vi "Autonomous Independent.vi"   [LabVIEW 2011]
doc: "This VI is called when autonomous begins, and will automatically be terminated when autonomous ends. You can carry out timed or sensor driven robot movement independently without needing to return to the caller."
uses:
  <vilib>/Rock Robotics/WPI/Solenoid/WPI_SolenoidValue.ctl
  Robot Global Data.vi
  <vilib>/Rock Robotics/WPI/Solenoid/WPI_SolenoidSetEnum.vi
types:
  T1 = typedef "WPI_RobotDriveDevRef.ctl" = cluster{"DevStatus":errorcluster, "Motors[]":T2[], "Square Inputs":bool, "Max Output":dbl, "Isochronous":bool}
  T2 = typedef "WPI_MotorControlDeviceRef.ctl" = cluster{"DeviceStatus":errorcluster, "Type":enum16{"PWM", "CAN"}, "PWM":cluster{"Digital Module":T3, "PWM Channel":T4, "DeadBand":T5}, "CAN":cluster{"Device Number":u8, "Control Mode":T6, "Semaphore":T7, "Max Vout":dbl}, "Invert":bool, "TransformRef":T8, "InvTransformRef":T8}
  T3 = typedef "FPGA_TypedefDigitalModule.ctl" = enum16{"Digital Module 1", "Digital Module 2"}
  T4 = typedef "FPGA_DIOPWMChannel.ctl" = enum8{"PWM 1", "PWM 2", "PWM 3", "PWM 4", "PWM 5", "PWM 6", "PWM 7", "PWM 8", "PWM 9", "PWM 10", "Invalid"}
  T5 = typedef "WPI_PWMDeadband.ctl" = cluster{"Name":string, "maxPositivePwm":i32, "minPositivePwm":i32, "centerPwm":i32, "maxNegativePwm":i32, "minNegativePwm":i32, "angularRange":u16}
  T6 = typedef "WPI_CANJaguar_ControlMode.ctl" = enum8{"Percent VBus", "Current", "Speed", "Position", "Voltage"}
  T7 = typedef "Semaphore RefNum" = refnum<k1>
  T8 = typedef "WPI_PWMTransform_ConPane.ctl" = refnum<vi>
  T9 = typedef "Autonomous Data.ctl" = cluster{"Auto Mode":enum16{"Do Nothing", "Shoot From Key", "Shoot From Key Center, Bridge", "Shoot From Key, Feed", "Shoot From Key, Drive Forward", "Fender From Center", "Fender From Right", "Fender From Left"}, "Delay (s)":dbl}
  T10 = typedef "WPI_GyroDevRef.ctl" = cluster{"DevStatus":errorcluster, "Analog Module":T11, "Analog Channel":T12, "Offset":dbl, "Gain (VoltsPerDegree/Second)":dbl}
  T11 = typedef "FPGA_TypedefAnalogModule.ctl" = enum16{"Analog Module 1", "Analog Module 2"}
  T12 = typedef "FPGA_AIChannel.ctl" = enum8{"AI 1", "AI 2", "AI 3", "AI 4", "AI 5", "AI 6", "AI 7", "AI 8", "Invalid"}
  T13 = enum16{"Do Nothing", "Shoot From Key", "Shoot From Key Center, Bridge", "Shoot From Key, Feed", "Shoot From Key, Drive Forward", "Fender From Center", "Fender From Right", "Fender From Left"}
  T14 = typedef "WPI_SolenoidValue.ctl" = enum16{"Off", "On", "Forward", "Reverse"}
  T15 = typedef "Position Typedef.ctl" = cluster{"X":dbl, "Y":dbl, "Heading":dbl}
  T16 = typedef "WPI_SolenoidDevRef.ctl" = cluster{"DevStatus":errorcluster, "Solenoid Module":T17, "Forward Solenoid Channel":T18, "Reverse Solenoid Channel":T18}
  T17 = typedef "FPGA_TypedefSolenoidModule.ctl" = enum16{"Solenoid Module 1", "Solenoid Module 2"}
  T18 = typedef "WPI_SolenoidChannel.ctl" = enum8{"Solenoid 1", "Solenoid 2", "Solenoid 3", "Solenoid 4", "Solenoid 5", "Solenoid 6", "Solenoid 7", "Solenoid 8", "Invalid"}
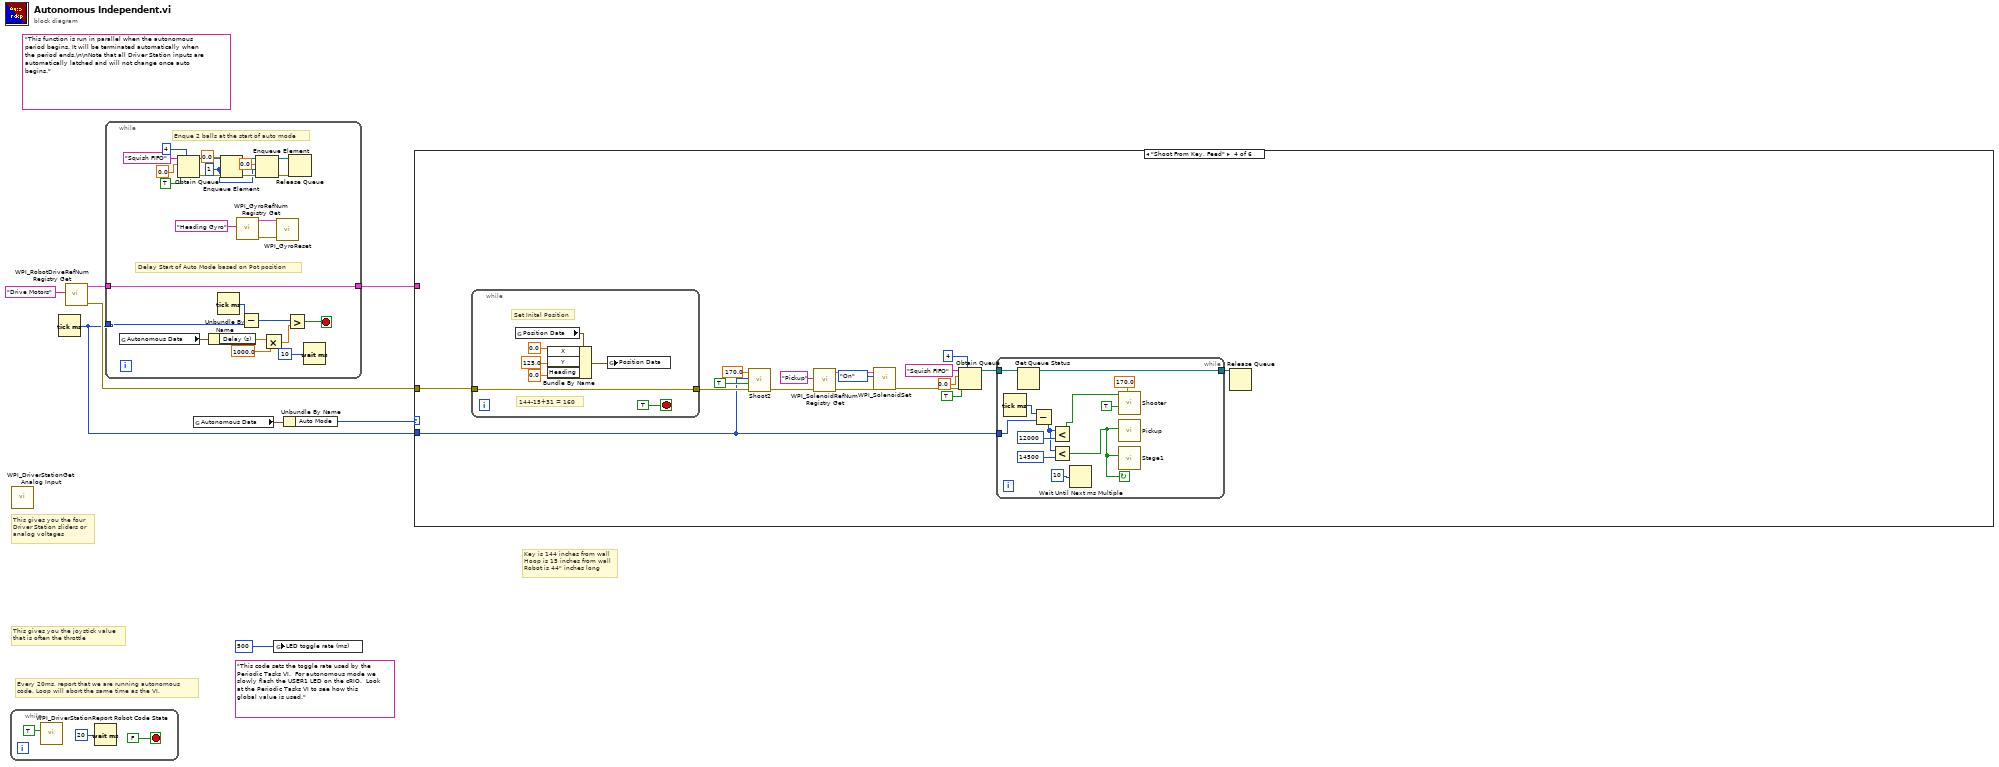
[diagram p0: block diagram]
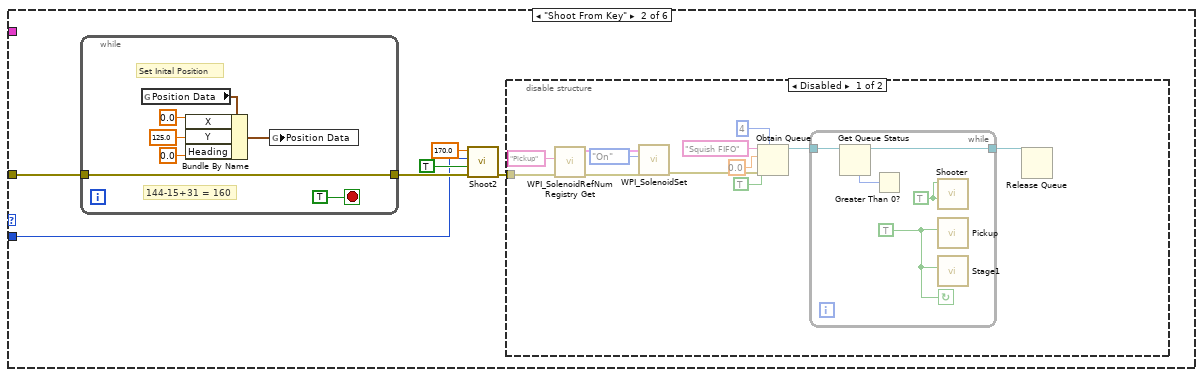
[diagram p3: hidden frame]
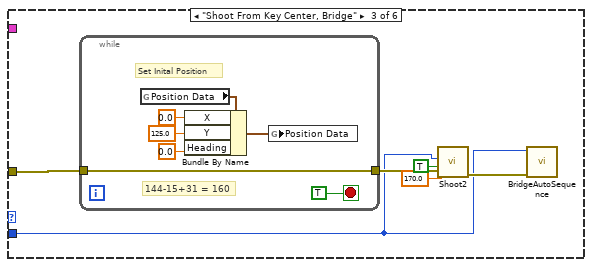
[diagram p5: hidden frame]
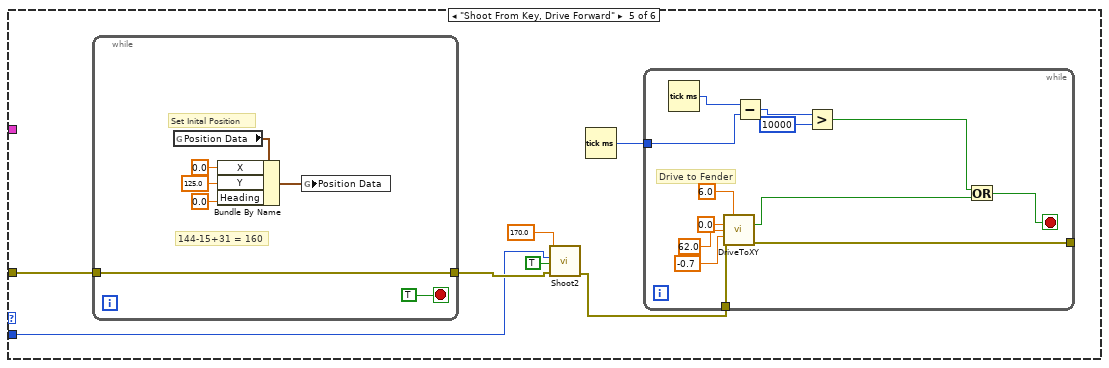
[diagram p6: hidden frame]
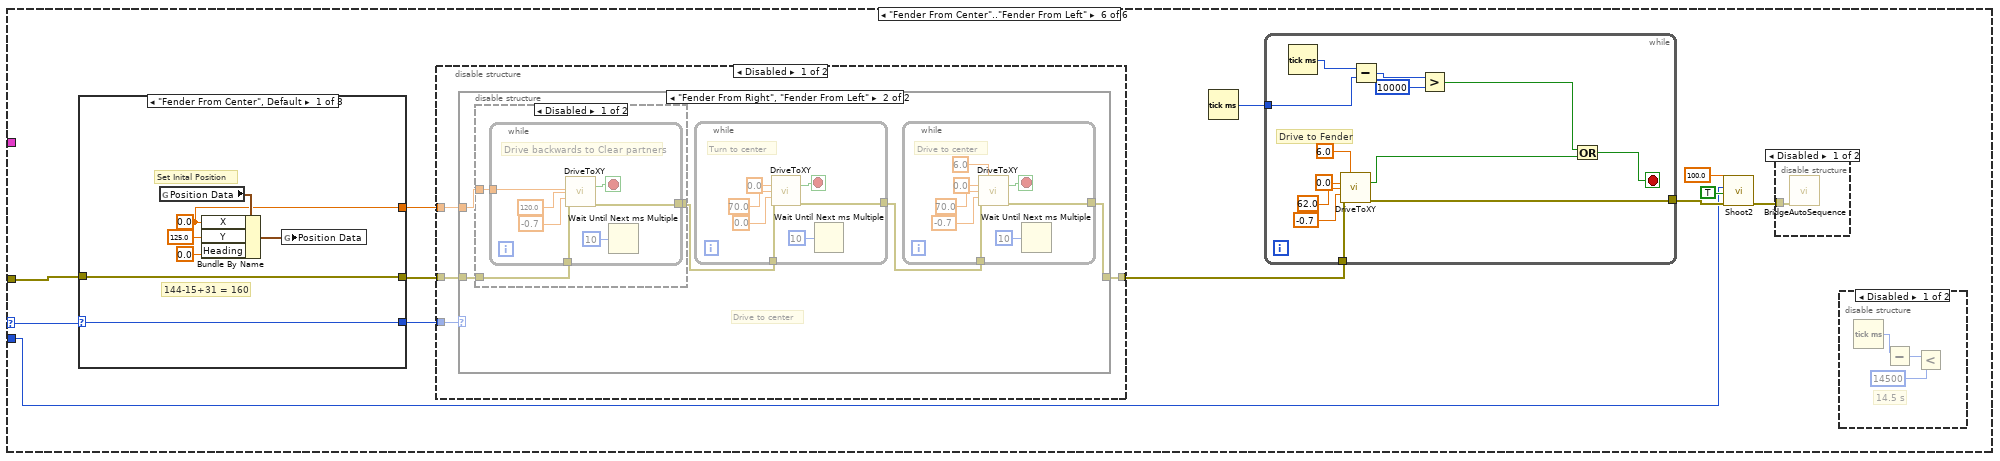
[diagram p7: hidden frame]
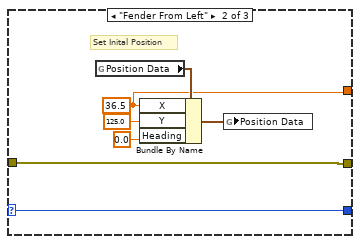
[diagram p13: hidden frame]
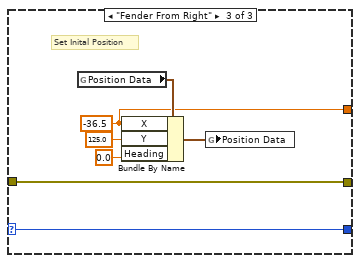
[diagram p14: hidden frame]
diagram:
  (unwired) "This code sets the toggle rate used by the Periodic Tasks VI.  For autonomous mode we slowly flash the USER1 LED on the cRIO.  Look at the Periodic Tasks VI to see how this global value is used."
  (unwired) "This function is run in parallel when the autonomous period begins. It will be terminated automatically when the period ends.\n\nNote that all Driver Station inputs are automatically latched and will not change once auto begins."
  # "Key is 144 inches from wall\nHoop is 15 inches from wall\nRobot is 44\" inches long"
  # "Every 20ms, report that we are running autonomous\ncode. Loop will abort the same time as the VI."
  # "This gives you the joystick value\nthat is often the throttle"
  # "This gives you the four\nDriver Station sliders or\nanalog voltages"
  n1 = while {
    stop <- FALSE stop-if-true
    n2 = call <vilib>:"WPI_DriverStationReport Robot Code State.vi"("Autonomous"=TRUE) -> ()  [unwired: 10 in, 1 out]
    n3 = Wait (ms)(milliseconds to wait=u32 20) -> ()  [unwired: 1 out]
  }
  n4 = call <vilib>:"WPI_DriverStationGet Analog Input.vi"() -> ()  [unwired: 12 out]
  n5 = Tick Count (ms)() -> (millisecond timer value=w1:u32)
  n6 = call <vilib>:"WPI_RobotDriveRefNum Registry Get.vi"("refnum name"="Drive Motors") -> ("error out"=w2:errorcluster, "RobotDriveDevRef"=w6:T1)  [unwired: 1 in, 8 out]
  n7 = while {
    tunnel: w1 -> [w36]
    tunnel: w6 -> [w33]
    tunnel: [w33] -> w3
    stop <- w35 stop-if-true
    w14 = 1 ("timeout in ms (-1)")
    # "Enque 2 balls at the start of auto mode"
    # "Delay Start of Auto Mode based on Pot position"
    n8 = global read "Robot Global Data.vi" "Autonomous Data"() -> (w31:T9)
    n9 = Obtain Queue(max queue size (-1, unlimited)=4, name (unnamed)="Squish FIFO", element data type=sgl 0.0 ("Voltage"), create if not found? (T)=TRUE) -> (queue out=w21:refnum<queue>, error out=w22:errorcluster)  [unwired: 1 in, 1 out]
    n10 = Unbundle By Name(w31) -> ("Delay (s)"=w29:dbl)
    n11 = Tick Count (ms)() -> (millisecond timer value=w32:u32)
    n12 = Enqueue Element(queue=w21, element=sgl 0.0, timeout in ms (-1)=w14, error in (no error)=w22) -> (queue out=w17:refnum<queue>, error out=w16:errorcluster)  [unwired: 1 out]
    n13 = call <vilib>:"WPI_GyroRefNum Registry Get.vi"("refnum name"="Heading Gyro") -> ("error out"=w26:errorcluster, "GyroDevRef"=w25:T10)  [unwired: 1 in, 8 out]
    n14 = Subtract(x=w32, y=w36) -> (x-y=w37:u32)
    n15 = Enqueue Element(queue=w17, element=sgl 0.0, timeout in ms (-1)=w14, error in (no error)=w16) -> (queue out=w12:refnum<queue>, error out=w13:errorcluster)  [unwired: 1 out]
    n16 = Multiply(x=w29, y=1000.0) -> (x*y=w30:dbl)
    n17 = call <vilib>:"WPI_GyroReset.vi"("error in (no error)"=w26, "GyroDevRef"=w25) -> ()  [unwired: 8 in, 2 out]
    n18 = Greater?(x=w37, y=w30) -> (0:w35:bool)
    n19 = Release Queue(queue=w12, error in (no error)=w13) -> ()  [unwired: 1 in, 3 out]
    n20 = Wait (ms)(milliseconds to wait=u32 10) -> ()  [unwired: 1 out]
  }
  n21 = global read "Robot Global Data.vi" "Autonomous Data"() -> (w5:T9)
  n22 = global write "Robot Global Data.vi" "LED toggle rate (ms)"(u32 500 ("LED ms toggle rate")) -> ()
  n23 = Unbundle By Name(w5) -> ("Auto Mode"=w4:T13)
  n24 = case shown="\"Shoot From Key, Feed\"" w4 {
    selector: w4 -> [_ _ _ _ _ w155]
    tunnel: w3 -> [_ _ _ _ _ _]
    tunnel: w2 -> [_ w43 w73 w94 w121 w154]
    tunnel: w1 -> [_ w39 w69 w81 w117 w145]
    frame "Do Nothing", Default {
    }
    frame "Shoot From Key" {
      n25 = while {
        tunnel: w43 -> [w64]
        tunnel: [w64] -> w42
        stop <- TRUE stop-if-true
        # "144-15+31 = 160"
        # "Set Inital Position"
        n26 = global read "Robot Global Data.vi" "Position Data"() -> (w67:T15)
        n27 = Bundle By Name(cluster=w67, "X"=0.0, "Y"=125.0, "Heading"=0.0) -> (w66:T15)
        n28 = global write "Robot Global Data.vi" "Position Data"(w66) -> ()
      }
      n29 = call "Shoot2.vi"("error in (no error)"=w42, "Use Camera"=TRUE, "Auto Start"=w39, "Distance"=170.0) -> ("error out"=w41:errorcluster)  [unwired: 7 in]
      n30 = disable-structure shown="Disabled" {
        disable-tunnel: w41 -> [w47 _]
        frame Disabled {
          n31 = call <vilib>:"WPI_SolenoidRefNum Registry Get.vi"("error in (no error)"=w47, "refnum name"="Pickup") -> ("error out"=w51:errorcluster, "SolenoidDevRef"=w49:T16)  [unwired: 8 in]
          n32 = call-poly <vilib>:"WPI_SolenoidSet.vi"("error in (no error)"=w51, "Value"=WPI_SolenoidValue."On", "SolenoidDevRef"=w49) -> ("error out"=w46:errorcluster)  [unwired: 7 in, 1 out]
          n33 = Obtain Queue(max queue size (-1, unlimited)=4, name (unnamed)="Squish FIFO", element data type=sgl 0.0 ("Voltage"), create if not found? (T)=TRUE, error in (no error)=w46) -> (queue out=w52:refnum<queue>)  [unwired: 2 out]
          n34 = while {
            tunnel: w52 -> [w58]
            tunnel: [w57] -> w45
            stop <- w60 continue-if-true
            w56 = TRUE ("Use Camera")
            w60 = TRUE ("Fire")
            n35 = Get Queue Status(queue=w58) -> (queue out=w57:refnum<queue>, # elements in queue=w59:i32)  [unwired: 2 in, 6 out]
            n36 = Greater Than 0?(x=w59) -> ()  [unwired: 1 out]
            n37 = call "Shooter.vi"("Use Camera"=w56, "Fire"=w56) -> ()  [unwired: 8 in, 2 out]
            n38 = call "Pickup.vi"("On?"=w60) -> ()  [unwired: 11 in]
            n39 = call "Stage1.vi"("On?"=w60) -> ()  [unwired: 11 in]
          }
          n40 = Release Queue(queue=w45) -> ()  [unwired: 2 in, 3 out]
        }
        frame Enabled {
        }
      }
    }
    frame "Shoot From Key Center, Bridge" {
      n41 = while {
        tunnel: w73 -> [w77]
        tunnel: [w77] -> w72
        stop <- TRUE stop-if-true
        # "144-15+31 = 160"
        # "Set Inital Position"
        n42 = global read "Robot Global Data.vi" "Position Data"() -> (w80:T15)
        n43 = Bundle By Name(cluster=w80, "X"=0.0, "Y"=125.0, "Heading"=0.0) -> (w79:T15)
        n44 = global write "Robot Global Data.vi" "Position Data"(w79) -> ()
      }
      n45 = call "Shoot2.vi"("error in (no error)"=w72, "Use Camera"=TRUE, "Auto Start"=w69, "Distance"=170.0) -> ("error out"=w71:errorcluster)  [unwired: 7 in]
      n46 = call "BridgeAutoSequence.vi"("error in (no error)"=w71, "Auto Start"=w69) -> ()  [unwired: 10 in]
    }
    frame "Shoot From Key, Feed" {
      n47 = while {
        tunnel: w94 -> [w113]
        tunnel: [w113] -> w97
        stop <- TRUE stop-if-true
        # "144-15+31 = 160"
        # "Set Inital Position"
        n48 = global read "Robot Global Data.vi" "Position Data"() -> (w116:T15)
        n49 = Bundle By Name(cluster=w116, "X"=0.0, "Y"=125.0, "Heading"=0.0) -> (w115:T15)
        n50 = global write "Robot Global Data.vi" "Position Data"(w115) -> ()
      }
      n51 = call "Shoot2.vi"("error in (no error)"=w97, "Use Camera"=TRUE, "Auto Start"=w81, "Distance"=170.0) -> ("error out"=w82:errorcluster)  [unwired: 7 in]
      n52 = call <vilib>:"WPI_SolenoidRefNum Registry Get.vi"("error in (no error)"=w82, "refnum name"="Pickup") -> ("error out"=w89:errorcluster, "SolenoidDevRef"=w87:T16)  [unwired: 8 in]
      n53 = call-poly <vilib>:"WPI_SolenoidSet.vi"("error in (no error)"=w89, "Value"=WPI_SolenoidValue."On", "SolenoidDevRef"=w87) -> ("error out"=w85:errorcluster)  [unwired: 7 in, 1 out]
      n54 = Obtain Queue(max queue size (-1, unlimited)=4, name (unnamed)="Squish FIFO", element data type=sgl 0.0 ("Voltage"), create if not found? (T)=TRUE, error in (no error)=w85) -> (queue out=w90:refnum<queue>)  [unwired: 2 out]
      n55 = while {
        tunnel: w90 -> [w109]
        tunnel: [w108] -> w84
        tunnel: w81 -> [w103]
        stop <- w98 continue-if-true
        n56 = Tick Count (ms)() -> (millisecond timer value=w104:u32)
        n57 = Get Queue Status(queue=w109) -> (queue out=w108:refnum<queue>)  [unwired: 2 in, 7 out]
        n58 = Subtract(x=w104, y=w103) -> (x-y=w100:u32)
        n59 = Less?(x=w100, y=u32 12000) -> (x < y?=w101:bool)
        n60 = Less?(x=w100, y=u32 14500) -> (x < y?=w98:bool)
        n61 = Wait Until Next ms Multiple(millisecond multiple=u32 10) -> ()  [unwired: 1 out]
        n62 = call "Shooter.vi"("Distance"=170.0, "Use Camera"=TRUE, "Fire"=w101) -> ()  [unwired: 7 in, 2 out]
        n63 = call "Pickup.vi"("On?"=w98) -> ()  [unwired: 11 in]
        n64 = call "Stage1.vi"("On?"=w98) -> ()  [unwired: 11 in]
      }
      n65 = Release Queue(queue=w84) -> ()  [unwired: 2 in, 3 out]
    }
    frame "Shoot From Key, Drive Forward" {
      n66 = while {
        tunnel: w121 -> [w124]
        tunnel: [w124] -> w119
        stop <- TRUE stop-if-true
        # "144-15+31 = 160"
        # "Set Inital Position"
        n67 = global read "Robot Global Data.vi" "Position Data"() -> (w129:T15)
        n68 = Bundle By Name(cluster=w129, "X"=0.0, "Y"=125.0, "Heading"=0.0) -> (w128:T15)
        n69 = global write "Robot Global Data.vi" "Position Data"(w128) -> ()
      }
      n70 = call "Shoot2.vi"("error in (no error)"=w119, "Use Camera"=TRUE, "Auto Start"=w117, "Distance"=170.0) -> ("error out"=w118:errorcluster)  [unwired: 7 in]
      n71 = Tick Count (ms)() -> (millisecond timer value=w122:u32)
      n72 = while {
        tunnel: [w141] -> _
        tunnel: w118 -> [w140]
        tunnel: w122 -> [w137]
        stop <- w132 stop-if-true
        # "Drive to Fender"
        n73 = Tick Count (ms)() -> (millisecond timer value=w138:u32)
        n74 = call "DriveToXY.vi"("Drive Margin"=6.0, "X Target"=0.0, "Y Target"=62.0, "Speed"=-0.7, "error in"=w140) -> ("At Target"=w134:bool, "error out"=w141:errorcluster)  [unwired: 8 in, 1 out]
        n75 = Subtract(x=w138, y=w137) -> (x-y=w136:u32)
        n76 = Greater?(x=w136, y=u32 10000) -> (0:w133:bool)
        n77 = Or(x=w133, y=w134) -> (x .or. y?=w132:bool)
      }
    }
    frame "Fender From Center".."Fender From Left" {
      n78 = case shown="\"Fender From Center\", Default" w155 {
        selector: w155 -> [w208 w215 w223]
        tunnel: w154 -> [w210 w217 w224]
        tunnel: [w210 w217 w224] -> w153
        tunnel: [w209 w216 w222] -> w152
        tunnel: [w208 w215 w223] -> w150
        frame "Fender From Center", Default {
          w209 = 0.0 ("X")
          # "144-15+31 = 160"
          # "Set Inital Position"
          n79 = global read "Robot Global Data.vi" "Position Data"() -> (w214:T15)
          n80 = Bundle By Name(cluster=w214, "X"=w209, "Y"=125.0, "Heading"=0.0) -> (w213:T15)
          n81 = global write "Robot Global Data.vi" "Position Data"(w213) -> ()
        }
        frame "Fender From Left" {
          w216 = 36.5 ("X")
          # "Set Inital Position"
          n82 = global read "Robot Global Data.vi" "Position Data"() -> (w221:T15)
          n83 = Bundle By Name(cluster=w221, "X"=w216, "Y"=125.0, "Heading"=0.0) -> (w220:T15)
          n84 = global write "Robot Global Data.vi" "Position Data"(w220) -> ()
        }
        frame "Fender From Right" {
          w222 = -36.5 ("X")
          # "Set Inital Position"
          n85 = global read "Robot Global Data.vi" "Position Data"() -> (w228:T15)
          n86 = Bundle By Name(cluster=w228, "X"=w222, "Y"=125.0, "Heading"=0.0) -> (w227:T15)
          n87 = global write "Robot Global Data.vi" "Position Data"(w227) -> ()
        }
      }
      n88 = disable-structure shown="Disabled" {
        disable-tunnel: w153 -> [w159 _]
        disable-tunnel: w152 -> [w158 _]
        disable-tunnel: [w157 _] -> w151
        disable-tunnel: w150 -> [w156 _]
        frame Disabled {
          n89 = case shown="\"Fender From Right\", \"Fender From Left\"" w156 {
            tunnel: w159 -> [w160 w164]
            tunnel: w158 -> [_ w165]
            tunnel: [w160 w161] -> w157
            frame "Do Nothing", Default {
            }
            frame "Fender From Right", "Fender From Left" {
              # "Drive to center"
              n90 = disable-structure shown="Disabled" {
                disable-tunnel: w165 -> [w168 _]
                disable-tunnel: w164 -> [w167 _]
                disable-tunnel: [w166 _] -> w163
                frame Disabled {
                  n91 = while {
                    tunnel: [w173] -> w166
                    tunnel: w167 -> [w172]
                    tunnel: w168 -> [w169]
                    stop <- w171 stop-if-true
                    # "Drive backwards to Clear partners"
                    n92 = call "DriveToXY.vi"("X Target"=w169, "Y Target"=120.0, "Speed"=-0.7, "error in"=w172) -> ("At Target"=w171:bool, "error out"=w173:errorcluster)  [unwired: 9 in, 1 out]
                    n93 = Wait Until Next ms Multiple(millisecond multiple=u32 10) -> ()  [unwired: 1 out]
                  }
                }
                frame Enabled {
                }
              }
              n94 = while {
                tunnel: [w188] -> w162
                tunnel: w163 -> [w187]
                stop <- w186 stop-if-true
                # "Turn to center"
                n95 = call "DriveToXY.vi"("X Target"=0.0, "Y Target"=70.0, "Speed"=0.0, "error in"=w187) -> ("At Target"=w186:bool, "error out"=w188:errorcluster)  [unwired: 9 in, 1 out]
                n96 = Wait Until Next ms Multiple(millisecond multiple=u32 10) -> ()  [unwired: 1 out]
              }
              n97 = while {
                tunnel: [w181] -> w161
                tunnel: w162 -> [w180]
                stop <- w179 stop-if-true
                # "Drive to center"
                n98 = call "DriveToXY.vi"("Drive Margin"=6.0, "X Target"=0.0, "Y Target"=70.0, "Speed"=-0.7, "error in"=w180) -> ("At Target"=w179:bool, "error out"=w181:errorcluster)  [unwired: 8 in, 1 out]
                n99 = Wait Until Next ms Multiple(millisecond multiple=u32 10) -> ()  [unwired: 1 out]
              }
            }
          }
        }
        frame Enabled {
        }
      }
      n100 = Tick Count (ms)() -> (millisecond timer value=w146:u32)
      n101 = while {
        tunnel: [w205] -> w148
        tunnel: w151 -> [w204]
        tunnel: w146 -> [w201]
        stop <- w196 stop-if-true
        # "Drive to Fender"
        n102 = Tick Count (ms)() -> (millisecond timer value=w202:u32)
        n103 = call "DriveToXY.vi"("Drive Margin"=6.0, "X Target"=0.0, "Y Target"=62.0, "Speed"=-0.7, "error in"=w204) -> ("At Target"=w198:bool, "error out"=w205:errorcluster)  [unwired: 8 in, 1 out]
        n104 = Subtract(x=w202, y=w201) -> (x-y=w200:u32)
        n105 = Greater?(x=w200, y=u32 10000) -> (0:w197:bool)
        n106 = Or(x=w197, y=w198) -> (x .or. y?=w196:bool)
      }
      n107 = call "Shoot2.vi"("error in (no error)"=w148, "Use Camera"=TRUE, "Auto Start"=w145, "Distance"=100.0) -> ("error out"=w149:errorcluster)  [unwired: 7 in]
      n108 = disable-structure shown="Disabled" {
        disable-tunnel: w149 -> [w191 _]
        frame Disabled {
          n109 = call "BridgeAutoSequence.vi"("error in (no error)"=w191) -> ()  [unwired: 11 in]
        }
        frame Enabled {
        }
      }
      n110 = disable-structure shown="Disabled" {
        frame Disabled {
          # "14.5 s"
          n111 = Tick Count (ms)() -> (millisecond timer value=w193:u32)
          n112 = Subtract(x=w193) -> (x-y=w192:u32)  [unwired: 1 in]
          n113 = Less?(x=w192, y=u32 14500) -> ()  [unwired: 1 out]
        }
        frame Enabled {
        }
      }
    }
  }
